vi "Read_Gripper_State.vi"(0 "error in":errorcluster, 2 "Side":T2, 3 "node":string) -> (1 "error out":errorcluster, 4 "EndEffectorState":T1)   [LabVIEW 2012]
doc: "Returns information from subscription to /sdk/robot/limb/<limb>/accessory/gripper/state"
uses:
  <userlib>/ROSforLV/ROS/Code/SubVIs/BaxterSide.ctl
  <userlib>/ROSforLV/ROS/Code/Console/Servers/ServerSubs/TopicDef.ctl
  <userlib>/ROSforLV/ROS/Code/SubVIs/_ROSDirection.ctl
panel:
  out "Reply":string
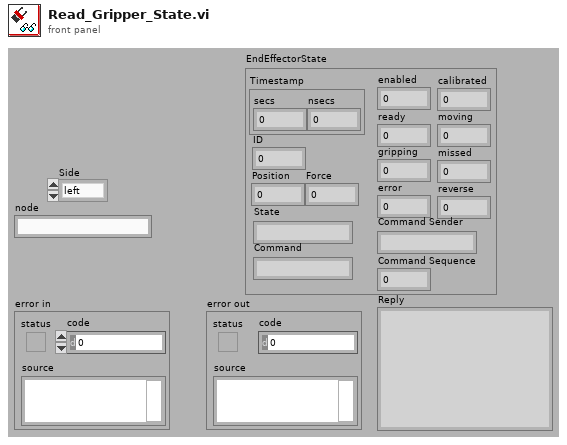
[diagram p1: front panel]
types:
  T1 = cluster{"Timestamp":cluster{"secs":i32, "nsecs":i32}, "ID":u32, "enabled":u8, "calibrated":u8, "ready":u8, "moving":u8, "gripping":u8, "missed":u8, "error":u8, "reverse":u8, "Position":sgl, "Force":sgl, "State":string, "Command":string, "Command Sender":string, "Command Sequence":u32}
  T2 = typedef "BaxterSide.ctl" = enum16{"left", "right"}
  T3 = typedef "TopicDef.ctl" = cluster{"Topic":string, "Type":string, "Action":T4, "Update (ms)":u16, "queue size":u16}
  T4 = typedef "_ROSDirection.ctl" = enum16{"Node", "Publisher", "Subscriber", "ServiceClient", "ServiceProvider"}
  T5 = typedef "_ROSControl.ctl" = cluster{"topic port":u16, "Node":string, "topic":string, "type":string, "node port":u16, "error ":errorcluster, "Direction":T4, "Update (ms)":u16, "FIFO size":u16}
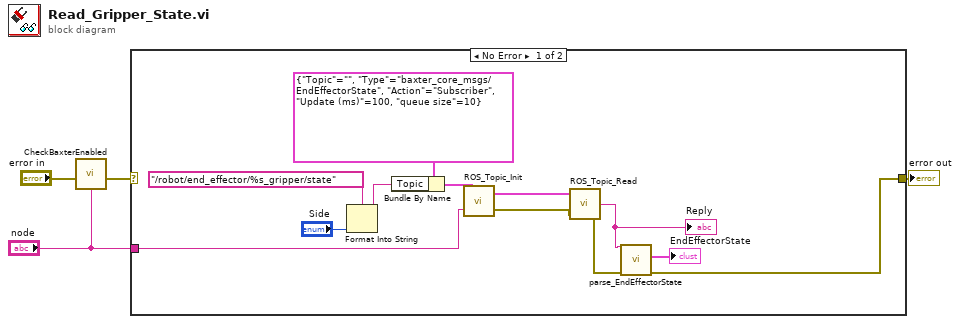
[diagram p0: block diagram]
diagram:
  n1 = call <userlib>:"CheckBaxterEnabled.vi"("error in"="error in", "node"="node") -> ("error out"=w2:errorcluster)  [unwired: 2 in]
  n2 = case shown="No Error" w2 {
    selector: w2 -> [_ w17]
    tunnel: [w5 w17] -> w4
    tunnel: "node" -> [w8 _]
    frame No Error {
      n3 = Format Into String(format string="/robot/end_effector/%s_gripper/state" ("Topic"), "Side") -> (resulting string=w14:string)  [unwired: 2 in, 1 out]
      n4 = Bundle By Name(cluster=T3 {"Topic"="", "Type"="baxter_core_msgs/EndEffectorState", "Action"=enum."Subscriber", "Update (ms)"=100, "queue size"=10} ("Definitions"), "Topic"=w14) -> (w11:T3)
      n5 = call <userlib>:"ROS_Topic_Init.vi"("node"=w8, "Definitions"=w11) -> ("error out"=w7:errorcluster, "ROS out"=w16:T5)
      n6 = call <userlib>:"ROS_Topic_Read.vi"("error in (no error)"=w7, "ROS in"=w16) -> ("error out"=w6:errorcluster, "Reply"=w10:string)  [unwired: 1 in, 1 out]
      "Reply" <- w10
      n7 = call <userlib>:"parse_EndEffectorState.vi"("error in"=w6, "msg in"=w10) -> ("error out"=w5:errorcluster, "EndEffectorState"=→"EndEffectorState":T1)  [unwired: 3 in, 1 out]
    }
    frame Error {
    }
  }
  "error out" <- w4
